vi "Shutdown.vi"(8 "error in (no error)":errorcluster) -> (0 "error out":errorcluster)   [LabVIEW 2023, in "Server.lvclass"]
uses:
  Server.lvclass
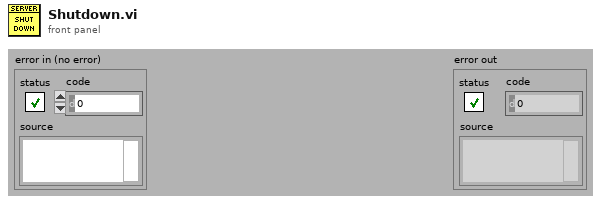
[diagram p1: front panel]
types:
  T1 = typedef "Server.lvclass/ObjectAttributes.ctl" = cluster{"Static Data":path, "MIME Types":variant, "Shutdown":bool, "API Queue":refnum<queue>, "ControlEndpoints":map{string, cluster{"Ref":refnum<vi>, "Mode":T2}}, "EventEndpoints":map{string, refnum<user-event>}}
  T2 = typedef "Control Ref Endpoint Access Mode.ctl" = enum16{"None", "Read/Write", "Read Only", "Write Only"}
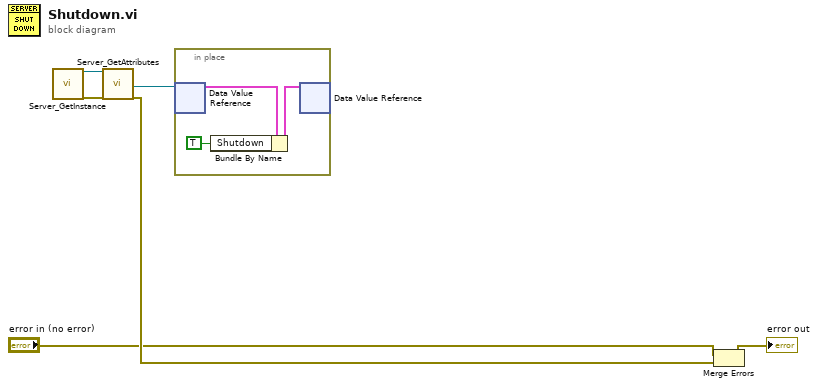
[diagram p0: block diagram]
diagram:
  n1 = call "Server_GetInstance.vi"() -> ("reference out"=w4:refnum<class "Server.lvclass">, "error out"=w5:errorcluster)  [unwired: 15 in, 3 out]
  n2 = call "Server_GetAttributes.vi"("reference in"=w4, "error in (no error)"=w5) -> ("DataRef"=w2:refnum<data-value>, "error out"=w3:errorcluster)  [unwired: 14 in, 2 out]
  n3 = in-place {
    n4 = in-place-dvr #1(w2) -> (w9:T1)  [unwired: 1 out]
    n5 = Bundle By Name(cluster=w9, "Shutdown"=TRUE) -> (w8:T1)
    n6 = in-place-dvr #1(w8) -> ()  [unwired: 2 out]
  }
  n7 = Merge Errors("error in (no error)", w3) -> (→"error out":errorcluster)
